vi "Dll 호출.vi"() -> ()   [LabVIEW 2014]
panel:
  out "반환 타입":i32
  out "randomArray":dbl[](array[numeric])
  in  "filePath":string
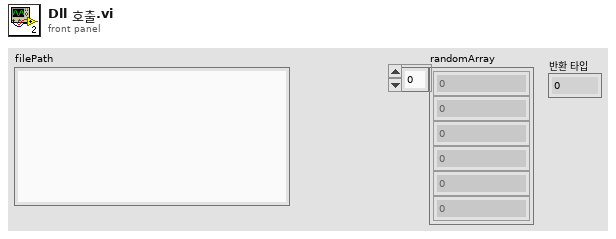
[diagram p1: front panel]
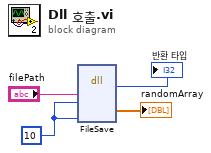
[diagram p0: block diagram]
diagram:
  w3 = 10 ("arraySize")
  n1 = dll-call lib="PTH2eabs CUserslveduDesktop중급 LabVIEW 실습builds\nDLL 생성\n나의 DLLLVSaveFile.dll" fn="FileSave"("filePath"="filePath", "arraySize"=w3, "len"=w3) -> ("반환 타입"=→"반환 타입":i32, "randomArray"=→"randomArray":dbl[])  [unwired: 7 in, 2 out]
